vi "Get Signal Channels.vi"(9 "Signal Index":i32, 10 "LQObject Manifestation":u64, 11 "Signal Map":variant) -> (2 "Signal Channels":variant[](array[variant]), 3 "Dup. Signal Map":variant)   [LabVIEW 2014, in "LQ Core.lvlib" / "LQCoreEngine.lvclass"]
uses:
  LQCoreEngine.lvclass
panel:
  # "Copyright (c) 2016 Sze Howe Koh\n\nThis Source Code Form is subject to the terms of the Mozilla Public\nLicense, v. 2.0. If a copy of the MPL was not distributed with this\nfile, You can obtain one at http://mozilla.org/MPL/2.0/."
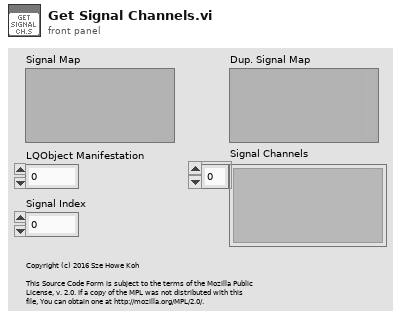
[diagram p1: front panel]
types:
  T1 = enum16{"big-endian, network order", "native, host order", "little-endian"}
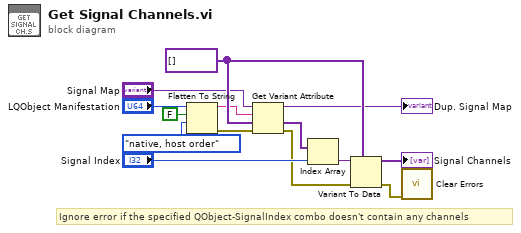
[diagram p0: block diagram]
diagram:
  w14 = variant[] []
  # "Ignore error if the specified QObject-SignalIndex combo doesn't contain any channels"
  n1 = Flatten To String(anything="LQObject Manifestation", prepend array or string size? (T)=FALSE, byte order (0:big-endian, network order)=T1."native, host order") -> (data string=w9:string, error out=w6:errorcluster)  [unwired: 1 in, 1 out]
  n2 = Get Variant Attribute(Variant="Signal Map", name=w9, default value (empty Variant)=w14, error in=w6) -> (duplicate Variant=→"Dup. Signal Map":variant, value=w3:variant[], error out=w1:errorcluster)  [unwired: 1 out]
  n3 = Index Array(array=w3, index="Signal Index") -> (element=w7:variant)
  n4 = Variant To Data(error in=w1, type=w14, Variant=w7) -> (data=→"Signal Channels":variant[], error out=w2:errorcluster)
  n5 = call <vilib>:"Clear Errors.vi"("error in (no error)"=w2) -> ()  [unwired: 5 in, 2 out]
